vi "Engine - Read Scanned Measurements.vi"(8 "error in (no error)":errorcluster, 9 "Output Channels Array In":dbl[](array[numeric]), 10 "DMM Ref In":refnum<k15>, 11 "Switch Ref In":refnum<k15>) -> (0 "error out":errorcluster, 1 "Output Channels Array Out":dbl[](array[numeric]), 2 "DMM Ref Out":refnum<k15>, 3 "Switch Ref Out":refnum<k15>)   [LabVIEW 2015, in "DMM-SWITCH-ScanList Engine.lvlib"]
doc: "Read hardware triggered scanned channels from the DMM and replace the Output Channels Array to send the measurements back to the VeriStand Engine."
uses:
  DMM-SWITCH-ScanList Engine.lvlib
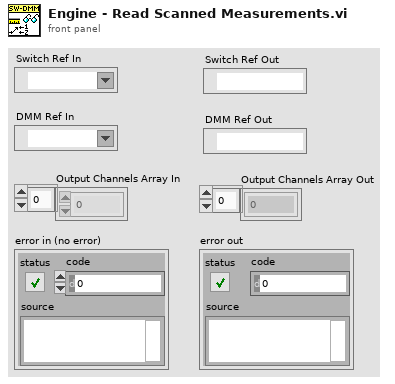
[diagram p1: front panel]
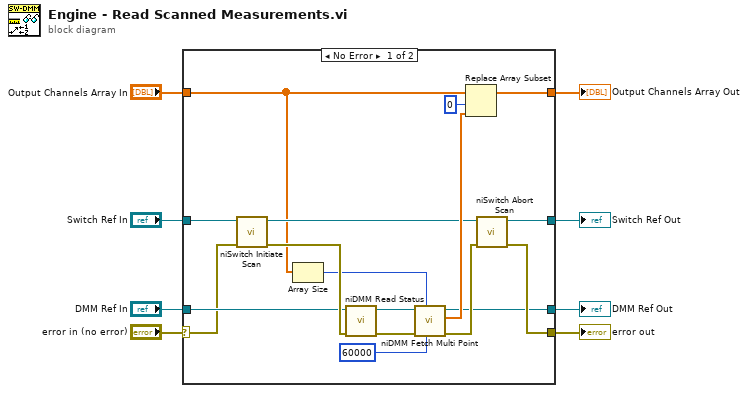
[diagram p0: block diagram]
diagram:
  n1 = case shown="No Error" "error in (no error)" {
    selector: "error in (no error)" -> [w13 w29]
    tunnel: "Output Channels Array In" -> [w10 w28]
    tunnel: [w24 w29] -> w7
    tunnel: "Switch Ref In" -> [w20 w27]
    tunnel: "DMM Ref In" -> [w15 w26]
    tunnel: [w14 w28] -> w4
    tunnel: [w12 w27] -> w1
    tunnel: [w11 w26] -> w2
    frame No Error {
      n2 = call <instrlib>:"niSwitch Initiate Scan.vi"("error in (no error)"=w13, "instrument handle"=w20) -> ("error out"=w21:errorcluster, "instrument handle out"=w23:refnum<k15>)  [unwired: 8 out]
      n3 = Array Size(array=w10) -> (size(s)=w9:i32)
      n4 = call <instrlib>:"niDMM Read Status.vi"("error in (no error)"=w21, "instrument handle"=w15) -> ("error out"=w18:errorcluster, "instrument handle out"=w17:refnum<k15>)  [unwired: 8 out]
      n5 = call <instrlib>:"niDMM Fetch Multi Point.vi"("Maximum Time (msec)"=60000, "Number to Fetch"=w9, "error in (no error)"=w18, "instrument handle"=w17) -> ("error out"=w22:errorcluster, "Measurements"=w25:dbl[], "instrument handle out"=w11:refnum<k15>)  [unwired: 5 out]
      n6 = Replace Array Subset(array=w10, new element=w25, index=0) -> (w14:dbl[])
      n7 = call <instrlib>:"niSwitch Abort Scan.vi"("error in (no error)"=w22, "instrument handle"=w23) -> ("error out"=w24:errorcluster, "instrument handle out"=w12:refnum<k15>)  [unwired: 8 out]
    }
    frame Error {
    }
  }
  "error out" <- w7
  "Output Channels Array Out" <- w4
  "Switch Ref Out" <- w1
  "DMM Ref Out" <- w2
